vi "Read Stage And Lasers Values.vi"(8 "error in (no error)":errorcluster, 9 "DataNotifier":refnum<notifier>[](array[refnum]), 10 "DataQueues":refnum<queue>[](array[refnum]), 11 "Config In":T1 {"Hardware Configuration"."Lasers Configuration"."SettingValues"."785 Power" format="%.1f"; "Hardware Configuration"."Lasers Configuration"."SettingValues"."647 Power" format="%.1f"; "Hardware Configuration"."Lasers Configuration"."SettingValues"."561 Power" format="%.1f"; "Hardware Configuration"."Lasers Configuration"."SettingValues"."532 Power" format="%.1f"; "Hardware Configuration"."Lasers Configuration"."SettingValues"."488 Power" format="%.1f"; "Hardware Configuration"."Lasers Configuration"."SettingValues"."405 Power" format="%.1f"}) -> (0 "error out":errorcluster)   [LabVIEW 2019]
uses:
  Settings/Settings.ctl
  Support/Hardware Configuration.ctl
  Support/Camera Configuration.ctl
  D:/SDK/PMQI-LabViewSamples/Examples/Dependencies/PVCamNET.dll
  <vilib>/userdefined/High Color/IMAQdx.ctl
  E:/DevHardSoftware/MMicroscopy/HardwareAdapter/Lasers/Dependencies/Oxxius_Boxx.dll
  Lasers/Dependencies/Oxxius_Boxx.dll
  Logging/Logging Configuration.ctl
  controls/UI Configuration.ctl
  controls/CallBack Refs.ctl
  Logging/Logging.lvlib
  Settings/Settings.lvlib
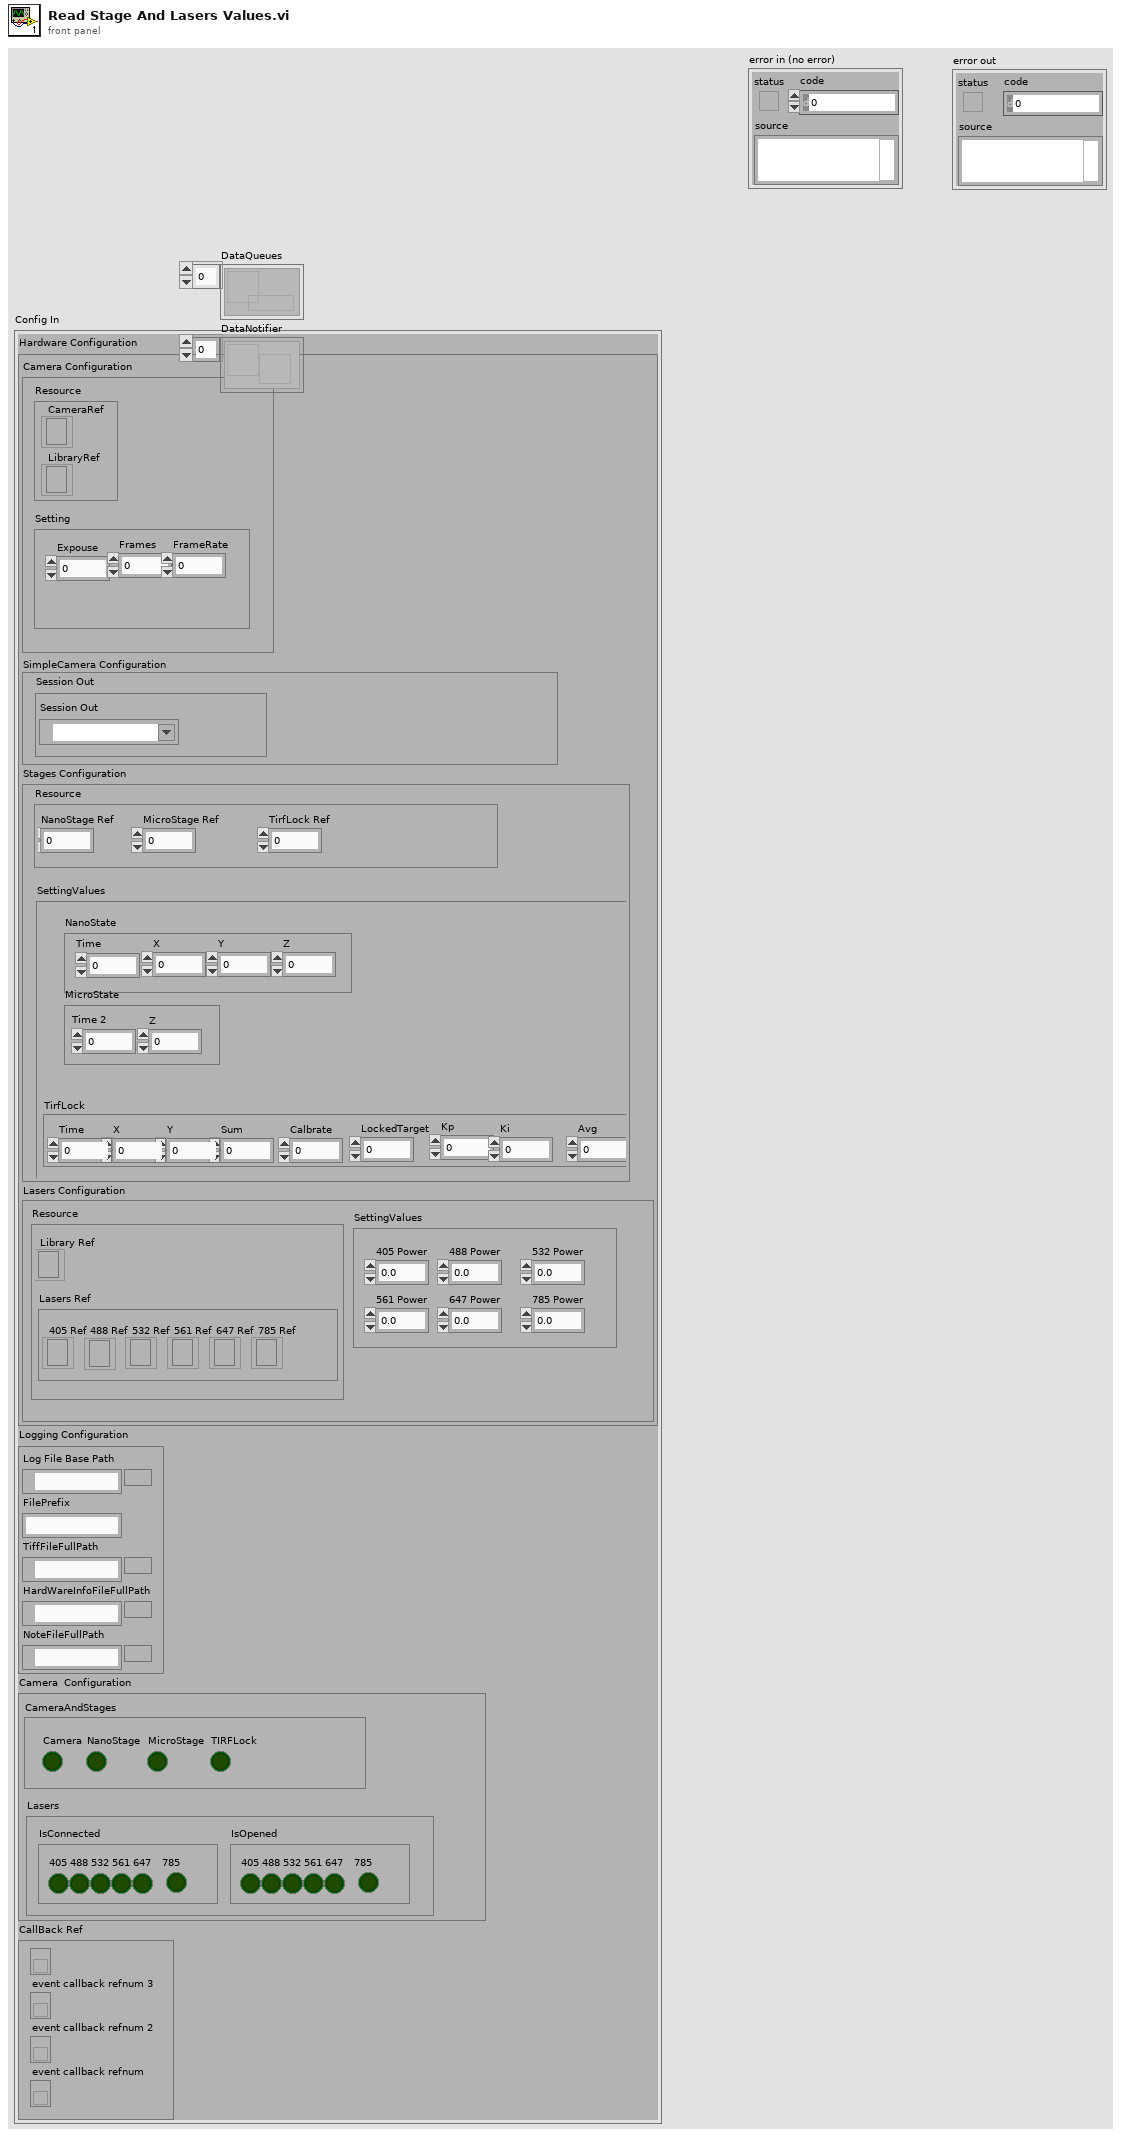
[diagram p1: front panel]
types:
  T1 = typedef "Settings.lvlib/Settings.ctl" = cluster{"Hardware Configuration":T2, "Logging Configuration":T5, "HardWare Status":cluster{"CameraAndStages":T6, "Lasers":cluster{"IsConnected":cluster{"405":bool, "488":bool, "532":bool, "561":bool, "647":bool, "785":bool}, "IsOpened":cluster{"405":bool, "488":bool, "532":bool, "561":bool, "647":bool, "785":bool}}}, "CallBack Ref":T7}
  T2 = typedef "Hardware Configuration.ctl" = cluster{"Camera Configuration":T3, "SimpleCamera Configuration":cluster{"Resource":cluster{"Session Out":T4}}, "Stages Configuration":cluster{"Resource":cluster{"NanoStage Ref":i32, "MicroStage Ref":i32, "TirfLock Ref":i32}, "SettingValues":cluster{"NanoState":cluster{"Time":dbl, "X":dbl, "Y":dbl, "Z":dbl}, "MicroState":cluster{"Time 2":dbl, "Z":dbl}, "TirfLock":cluster{"Time":dbl, "X":dbl, "Y":dbl, "Sum":dbl, "Calbrate":dbl, "LockedTarget":dbl, "Kp":dbl, "Ki":dbl, "Avg":dbl}}}, "Lasers Configuration":cluster{"SettingValues":cluster{"405 Power":sgl, "488 Power":sgl, "532 Power":sgl, "561 Power":sgl, "647 Power":sgl, "785 Power":sgl}, "Resource":cluster{"Library Ref":refnum<k24>, "Lasers Ref":cluster{"405 Ref":refnum<k24>, "488 Ref":refnum<k24>, "532 Ref":refnum<k24>, "561 Ref":refnum<k24>, "647 Ref":refnum<k24>, "785 Ref":refnum<k24>}}}}
  T3 = typedef "Camera Configuration.ctl" = cluster{"Resource":cluster{"CameraRef":refnum<k24>, "LibraryRef":refnum<k24>}, "Setting":cluster{"Expouse":dbl, "Frames":dbl, "FrameRate":dbl}}
  T4 = typedef "IMAQdx.ctl" = refnum<k21>
  T5 = typedef "Logging.lvlib/Logging Configuration.ctl" = cluster{"Log File Base Path":path, "FilePrefix":string, "TiffFileFullPath":path, "HardWareInfoFileFullPath":path, "NoteFileFullPath":path}
  T6 = typedef "UI Configuration.ctl" = cluster{"Camera":bool, "NanoStage":bool, "MicroStage":bool, "TIRFLock":bool}
  T7 = typedef "CallBack Refs.ctl" = cluster{"event callback refnum":refnum<k27>, "event callback refnum 2":refnum<k27>, "event callback refnum 3":refnum<k27>, "event callback refnum 4":refnum<k27>}
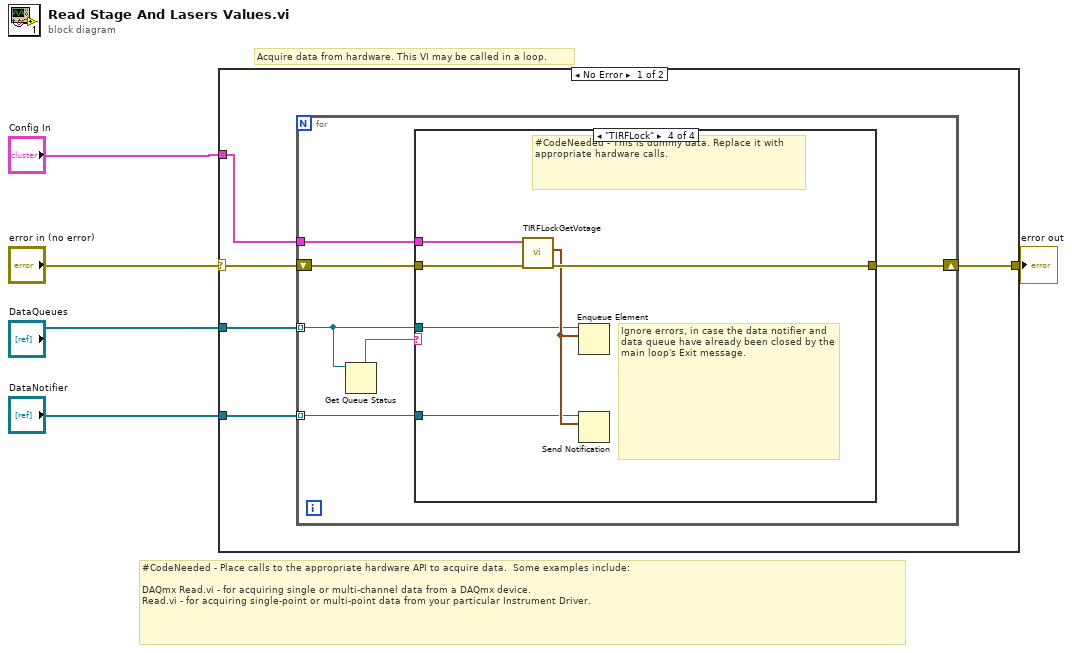
[diagram p0: block diagram]
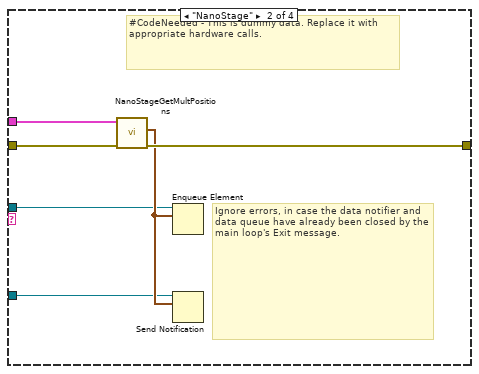
[diagram p3: hidden frame]
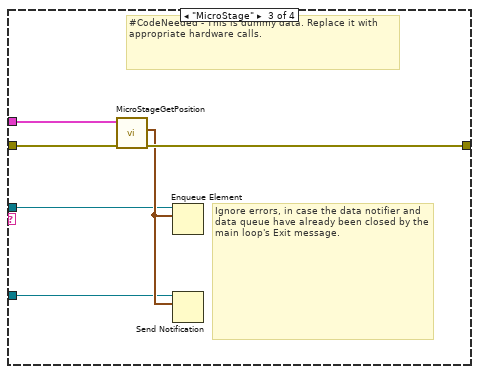
[diagram p4: hidden frame]
diagram:
  # "Acquire data from hardware. This VI may be called in a loop."
  # "#CodeNeeded - Place calls to the appropriate hardware API to acquire data.  Some examples include:\n\nDAQmx Read.vi - for acquiring single or multi-channel data from a DAQmx device.\nRead.vi - for acquiring single-point or multi-point data from your particular Instrument Driver."
  n1 = case shown="No Error" "error in (no error)" {
    selector: "error in (no error)" -> [w10 w36]
    tunnel: [w9 w36] -> w4
    tunnel: "DataNotifier" -> [w6 _]
    tunnel: "Config In" -> [w8 _]
    tunnel: "DataQueues" -> [w7 _]
    frame No Error {
      n2 = for {
        tunnel: w8 -> [w14]
        shift-right: [w15] -> w9
        shift-left: w10 -> [w16]
        tunnel: w7 -> [w12] mode=indexing
        tunnel: w6 -> [w13] mode=indexing
        n3 = Get Queue Status(queue=w12) -> (queue name=w11:string)  [unwired: 2 in, 7 out]
        n4 = case shown="\"TIRFLock\"" w11 {
          tunnel: w16 -> [w17 w23 w29 w35]
          tunnel: [w17 w22 w28 w34] -> w15
          tunnel: w14 -> [_ w21 w27 w33]
          tunnel: w13 -> [_ w19 w25 w31]
          tunnel: w12 -> [_ w18 w24 w30]
          frame Default {
          }
          frame "NanoStage" {
            # "Ignore errors, in case the data notifier and data queue have already been closed by the main loop's Exit message."
            # "#CodeNeeded - This is dummy data. Replace it with appropriate hardware calls."
            n5 = call "NanoStageGetMultPositions.vi"("error in (no error)"=w23, "Config In"=w21) -> ("error out"=w22:errorcluster, "Positions"=w20:cluster{"Time":dbl, "x":dbl, "y":dbl, "z":dbl})  [unwired: 6 in, 1 out]
            n6 = Enqueue Element(queue=w18, element=w20) -> ()  [unwired: 2 in, 3 out]
            n7 = Send Notification(notification=w20, notifier=w19) -> ()  [unwired: 1 in, 2 out]
          }
          frame "MicroStage" {
            # "Ignore errors, in case the data notifier and data queue have already been closed by the main loop's Exit message."
            # "#CodeNeeded - This is dummy data. Replace it with appropriate hardware calls."
            n8 = call "MicroStageGetPosition.vi"("error in (no error)"=w29, "Config In"=w27) -> ("error out"=w28:errorcluster, "Position"=w26:cluster{"Time":dbl, "z":dbl})  [unwired: 6 in, 1 out]
            n9 = Enqueue Element(queue=w24, element=w26) -> ()  [unwired: 2 in, 3 out]
            n10 = Send Notification(notification=w26, notifier=w25) -> ()  [unwired: 1 in, 2 out]
          }
          frame "TIRFLock" {
            # "Ignore errors, in case the data notifier and data queue have already been closed by the main loop's Exit message."
            # "#CodeNeeded - This is dummy data. Replace it with appropriate hardware calls."
            n11 = call "TIRFLockGetVotage.vi"("error in (no error)"=w35, "Config In"=w33) -> ("error out"=w34:errorcluster, "TirfLock"=w32:cluster{"Time":dbl, "X":dbl, "Y":dbl, "Sum":dbl})  [unwired: 6 in, 1 out]
            n12 = Enqueue Element(queue=w30, element=w32) -> ()  [unwired: 2 in, 3 out]
            n13 = Send Notification(notification=w32, notifier=w31) -> ()  [unwired: 1 in, 2 out]
          }
        }
      }
    }
    frame Error {
    }
  }
  "error out" <- w4
